vi "Vision Shooter Center.vi"(0 "Intake":dbl=1.0, 1 "X axis value":dbl=0.05 format="%#_13g", 2 "X axis value 2":dbl=-0.05) -> ()   [LabVIEW 2015]
uses:
  Robot Global Data.vi
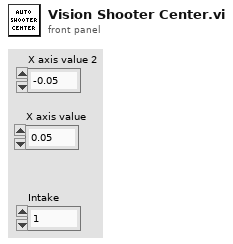
[diagram p1: front panel]
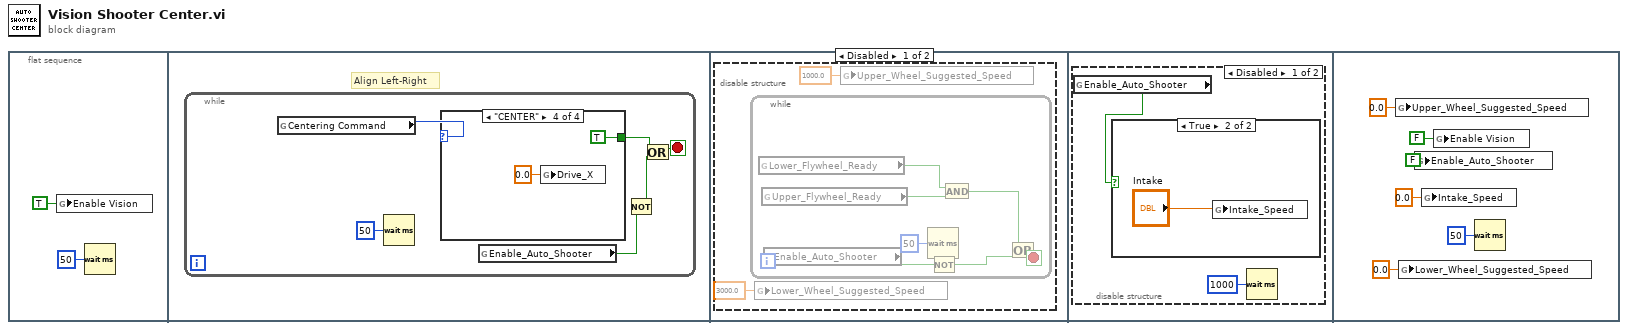
[diagram p0: block diagram]
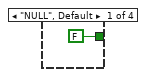
[diagram p2: hidden frame]
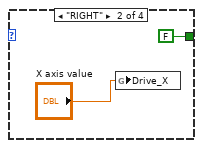
[diagram p3: hidden frame]
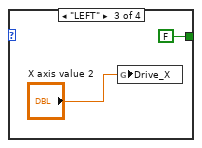
[diagram p4: hidden frame]
diagram:
  n1 = flat-sequence {
    frame #0 {
      n2 = global write "Robot Global Data.vi" "Enable Vision"(TRUE ("Enable Vision")) -> ()
      n3 = Wait (ms)(milliseconds to wait=u32 50) -> ()  [unwired: 1 out]
    }
    frame #1 {
      # "Align Left-Right"
      n4 = while {
        stop <- w5 stop-if-true
        n5 = global read "Robot Global Data.vi" "Centering Command"() -> (w7:enum16{"NULL", "RIGHT", "LEFT", "CENTER"})
        n6 = Wait (ms)(milliseconds to wait=u32 50) -> ()  [unwired: 1 out]
        n7 = case shown="\"CENTER\"" w7 {
          tunnel: [FALSE FALSE FALSE TRUE] -> w8
          frame "NULL", Default {
          }
          frame "RIGHT" {
            n8 = global write "Robot Global Data.vi" "Drive_X"("X axis value") -> ()
          }
          frame "LEFT" {
            n9 = global write "Robot Global Data.vi" "Drive_X"("X axis value 2") -> ()
          }
          frame "CENTER" {
            n10 = global write "Robot Global Data.vi" "Drive_X"(0.0 ("Drive_X")) -> ()
          }
        }
        n11 = global read "Robot Global Data.vi" "Enable_Auto_Shooter"() -> (w4:bool)
        n12 = Not(x=w4) -> (.not. x?=w3:bool)
        n13 = Or(x=w8, y=w3) -> (x .or. y?=w5:bool)
      }
    }
    frame #2 {
      n14 = disable-structure shown="Disabled" {
        frame Disabled {
          n15 = while {
            stop <- w20 stop-if-true
            n16 = global read "Robot Global Data.vi" "Lower_Flywheel_Ready"() -> (w23:bool)
            n17 = global read "Robot Global Data.vi" "Upper_Flywheel_Ready"() -> (w24:bool)
            n18 = global read "Robot Global Data.vi" "Enable_Auto_Shooter"() -> (w19:bool)
            n19 = Wait (ms)(milliseconds to wait=u32 50) -> ()  [unwired: 1 out]
            n20 = Not(x=w19) -> (.not. x?=w18:bool)
            n21 = And(x=w23, y=w24) -> (x .and. y?=w22:bool)
            n22 = Or(x=w22, y=w18) -> (x .or. y?=w20:bool)
          }
          n23 = global write "Robot Global Data.vi" "Lower_Wheel_Suggested_Speed"(3000.0 ("Lower_Wheel_Suggested_Speed")) -> ()
          n24 = global write "Robot Global Data.vi" "Upper_Wheel_Suggested_Speed"(1000.0 ("Upper_Wheel_Suggested_Speed")) -> ()
        }
        frame Enabled {
        }
      }
    }
    frame #3 {
      n25 = disable-structure shown="Disabled" {
        frame Disabled {
          n26 = global read "Robot Global Data.vi" "Enable_Auto_Shooter"() -> (w25:bool)
          n27 = case shown="True" w25 {
            frame False {
            }
            frame True {
              n28 = global write "Robot Global Data.vi" "Intake_Speed"("Intake") -> ()
            }
          }
          n29 = Wait (ms)(milliseconds to wait=u32 1000) -> ()  [unwired: 1 out]
        }
        frame Enabled {
        }
      }
    }
    frame #4 {
      n30 = global write "Robot Global Data.vi" "Upper_Wheel_Suggested_Speed"(0.0 ("Upper_Wheel_Suggested_Speed")) -> ()
      n31 = global write "Robot Global Data.vi" "Lower_Wheel_Suggested_Speed"(0.0 ("Lower_Wheel_Suggested_Speed")) -> ()
      n32 = global write "Robot Global Data.vi" "Enable_Auto_Shooter"(FALSE ("Enable_Shooter")) -> ()
      n33 = global write "Robot Global Data.vi" "Intake_Speed"(0.0 ("Intake_Speed")) -> ()
      n34 = global write "Robot Global Data.vi" "Enable Vision"(FALSE ("Enable Vision")) -> ()
      n35 = Wait (ms)(milliseconds to wait=u32 50) -> ()  [unwired: 1 out]
    }
  }
